vi "AddPrevious.vi"(10 "In":dbl) -> (2 "Out":dbl)   [LabVIEW 2020]
doc: "Simple example of use feedback node,"
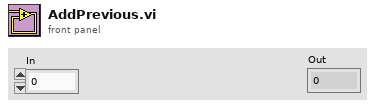
[diagram p1: front panel]
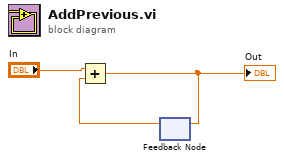
[diagram p0: block diagram]
diagram:
  n1 = feedback #1() -> (w2:dbl)  [unwired: 1 in]
  n2 = Add(x="In", y=w2) -> (x+y=w1:dbl)
  "Out" <- w1
  n3 = feedback-in #1(w1) -> ()
